vi "GT Get Fun Id.vi"(8 "error in (no error)":errorcluster caption="错误输入（无错误）", 9 "pFunId":i16, 10 "pFunName":string, 11 "cardNum":i16) -> (0 "error out":errorcluster caption="错误输出", 1 "pFunId out":i16, 2 "pFunName out":string, 3 "function return":i16)   [LabVIEW 2014, in "gts.lvlib"]
doc: "GT_API GT_GetFunId(short cardNum,char *pFunName,short *pFunId);"
uses:
  gts.lvlib
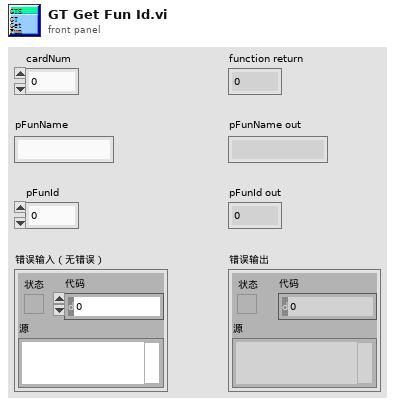
[diagram p1: front panel]
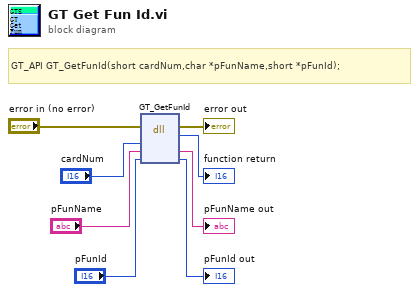
[diagram p0: block diagram]
diagram:
  # "GT_API GT_GetFunId(short cardNum,char *pFunName,short *pFunId);"
  n1 = dll-call lib="PTH2habs D固高科技资料GTS控制卡GTS卡18年上半年资料dllVC32bit\nmulti_cardgts.*" fn="GT_GetFunId"(error in="error in (no error)", "cardNum"="cardNum", "pFunName"="pFunName", "pFunId"="pFunId") -> (error out=→"error out":errorcluster, →"function return":i16, "pFunName"=→"pFunName out":string, "pFunId"=→"pFunId out":i16)  [unwired: 3 in, 1 out]
